vi "Find csv or xls.vi"(11 "String":string) -> (3 "Format":string)   [LabVIEW 2012]
panel:
  out "CSV":bool
  out "XLS":bool
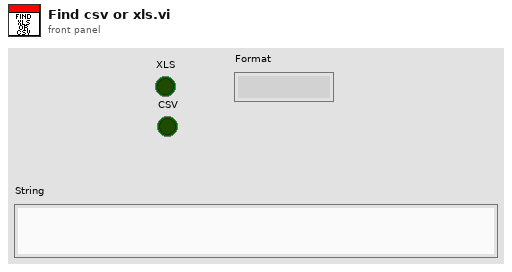
[diagram p1: front panel]
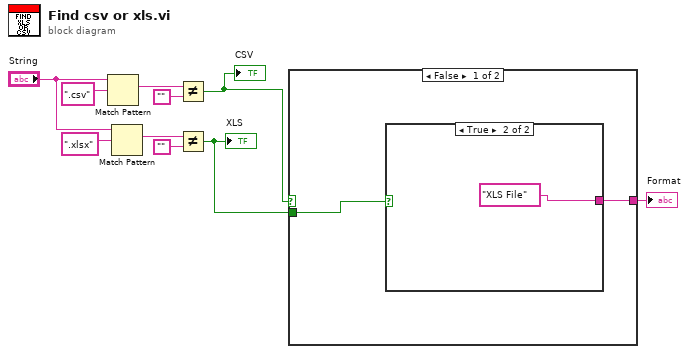
[diagram p0: block diagram]
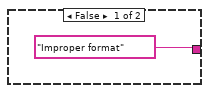
[diagram p2: hidden frame]
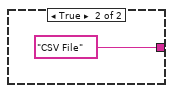
[diagram p3: hidden frame]
diagram:
  n1 = Match Pattern(string="String", regular expression=".csv") -> (match substring=w7:string)  [unwired: 1 in, 3 out]
  n2 = Match Pattern(string="String", regular expression=".xlsx") -> (match substring=w9:string)  [unwired: 1 in, 3 out]
  n3 = Not Equal?(x=w7, y="") -> (x != y?=w3:bool)
  "CSV" <- w3
  n4 = Not Equal?(x=w9, y="") -> (x != y?=w2:bool)
  "XLS" <- w2
  n5 = case shown="False" w3 {
    tunnel: [w11 "CSV File"] -> w1
    tunnel: w2 -> [w12 _]
    frame False {
      n6 = case shown="True" w12 {
        tunnel: ["Improper format" "XLS File"] -> w11
        frame False {
        }
        frame True {
        }
      }
    }
    frame True {
    }
  }
  "Format" <- w1
